vi "Darcy.vi"(6 "Density (kg/m^3)":dbl, 7 "Length (m)":dbl, 9 "Effective Diameter (m)":dbl, 10 "Velocity (m/s)":dbl, 11 "Friction Factor":dbl) -> (3 "Loss (Pa)":dbl)   [LabVIEW 2019]
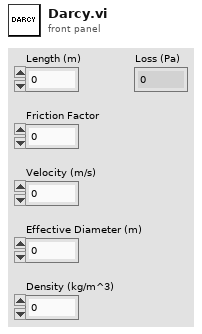
[diagram p1: front panel]
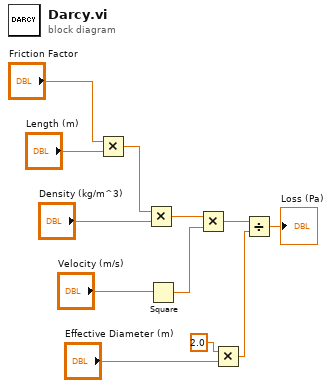
[diagram p0: block diagram]
diagram:
  n1 = Multiply(x="Friction Factor", y="Length (m)") -> (x*y=w2:dbl)
  n2 = Multiply(x=w2, y="Density (kg/m^3)") -> (x*y=w1:dbl)
  n3 = Square(x="Velocity (m/s)") -> (x^2=w7:dbl)
  n4 = Multiply(x=w1, y=w7) -> (x*y=w11:dbl)
  n5 = Multiply(x=2.0, y="Effective Diameter (m)") -> (x*y=w10:dbl)
  n6 = Divide(x=w11, y=w10) -> (x/y=→"Loss (Pa)":dbl)
